vi "edittest List Sequences.vi"(6 "User Information":T1, 8 "error in (no error)":errorcluster, 10 "sxSequenceId (\"\")":string, 11 "Connection Refnum":T2) -> (0 "error out":errorcluster, 2 "Sequences List":string, 3 "Connection Refnum":T2)   [LabVIEW 2011]
uses:
  Summitek EXT/ODBC/SQL Controls/Connection Refnum.ctl
  server/database/Users/User Record.ctl
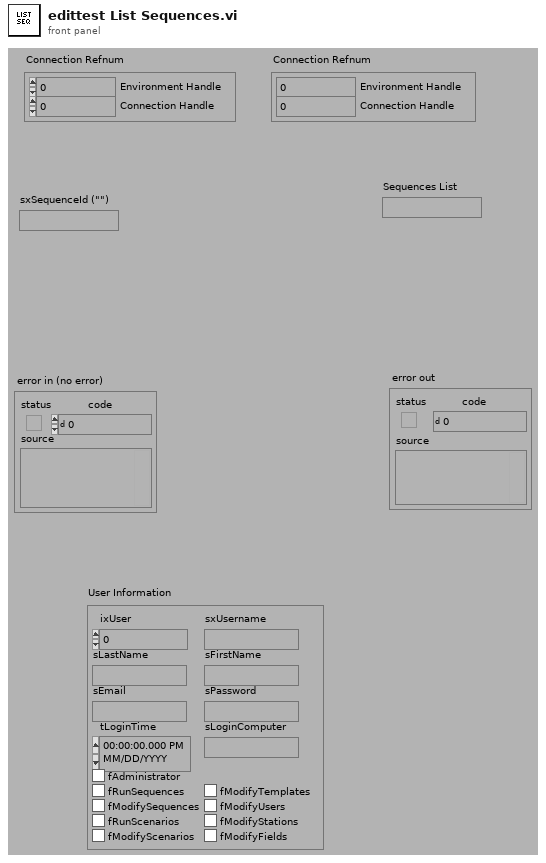
[diagram p1: front panel]
types:
  T1 = typedef "User Record.ctl" = cluster{"ixUser":i32, "sxUsername":string, "sLastName":string, "sFirstName":string, "sEmail":string, "sPassword":string, "tLoginTime":timestamp, "sLoginComputer":string, "fAdministrator":bool, "fRunSequences":bool, "fModifySequences":bool, "fRunScenarios":bool, "fModifyScenarios":bool, "fModifyTemplates":bool, "fModifyUsers":bool, "fModifyStations":bool, "fModifyFields":bool}
  T2 = typedef "Connection Refnum.ctl" = cluster{"Environment Handle":i32, "Connection Handle":i32}
  T3 = typedef "Sequence Record.ctl" = cluster{"ixSequence":i32, "sxSequenceId":string, "sDescription":string, "sCreator":string, "tCreationDate":timestamp, "sModifier":string, "tModifiedDate":timestamp, "fApproved":bool, "fSpartanSetsSN":bool, "fOverwriteData":bool, "fStopOnFail":bool, "fDisableQuickMode":bool, "fPartialExecution":bool, "fAutoNextItem":bool, "fDoNotPrintOnFail":bool}
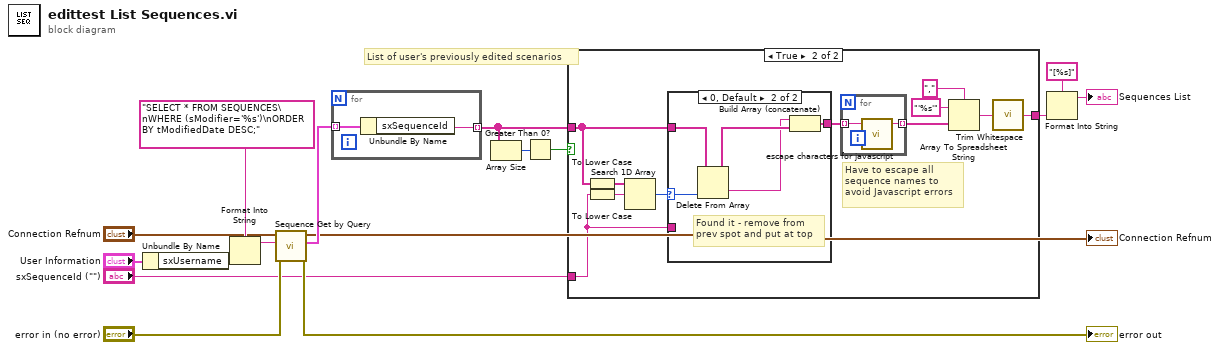
[diagram p0: block diagram]
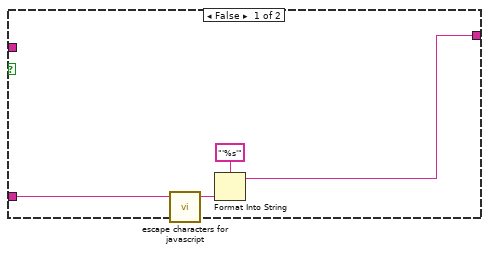
[diagram p2: hidden frame]
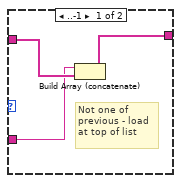
[diagram p3: hidden frame]
diagram:
  # "List of user's previously edited scenarios"
  n1 = Unbundle By Name("User Information") -> ("sxUsername"=w13:string)
  n2 = Format Into String(format string="SELECT * FROM SEQUENCES\nWHERE (sModifier='%s')\nORDER BY tModifiedDate DESC;", w13) -> (resulting string=w15:string)  [unwired: 2 in, 1 out]
  n3 = call "Sequence Get by Query.vi"("error in (no error)"="error in (no error)", "Sequence Query (\"\")"=w15, "Connection Refnum"="Connection Refnum") -> ("error out"=→"error out":errorcluster, "Records"=w14:T3[], "Connection Refnum"=→"Connection Refnum":T2)  [unwired: 6 out]
  n4 = for {
    tunnel: w14 -> [w18] mode=indexing
    tunnel: [w17] -> w2 mode=indexing
    n5 = Unbundle By Name(w18) -> ("sxSequenceId"=w17:string)
  }
  n6 = Array Size(array=w2) -> (size(s)=w6:i32)
  n7 = Greater Than 0?(x=w6) -> (x > 0?=w1:bool)
  n8 = case shown="True" w1 {
    tunnel: "sxSequenceId (\"\")" -> [w20 w25]
    tunnel: [w19 w27] -> w3
    tunnel: w2 -> [_ w26]
    frame False {
      n9 = call "escape characters for javascript.vi"("String (\"\")"=w20) -> ("escaped String"=w22:string)  [unwired: 4 out]
      n10 = Format Into String(format string="'%s'", w22) -> (resulting string=w19:string)  [unwired: 2 in, 1 out]
    }
    frame True {
      # "Have to escape all sequence names to avoid Javascript errors"
      n11 = To Lower Case(string=w26) -> (all lower case string=w28:string[])
      n12 = To Lower Case(string=w25) -> (all lower case string=w30:string)
      n13 = Search 1D Array(1D array=w28, element=w30) -> (index of element=w29:i32)  [unwired: 1 out]
      n14 = case shown="0, Default" w29 {
        selector: w29 -> [_ w42]
        tunnel: w26 -> [w38 w43]
        tunnel: w25 -> [w37 _]
        tunnel: [w36 w40] -> w23
        frame ..-1 {
          # "Not one of \nprevious - load\nat top of list"
          n15 = Build Array (concatenate)(w37, w38) -> (w36:string[])
        }
        frame 0, Default {
          # "Found it - remove from\nprev spot and put at top"
          n16 = Delete From Array(array=w43, index=w42) -> (deleted portion=w39:string, array with subset deleted=w41:string[])  [unwired: 1 in]
          n17 = Build Array (concatenate)(w39, w41) -> (w40:string[])
        }
      }
      n18 = for {
        tunnel: [w35] -> w24 mode=indexing
        tunnel: w23 -> [w34] mode=indexing
        n19 = call "escape characters for javascript.vi"("String (\"\")"=w34) -> ("escaped String"=w35:string)  [unwired: 4 out]
      }
      n20 = Array To Spreadsheet String(delimiter (Tab)=",", array=w24, 3:"'%s'") -> (spreadsheet string=w31:string)
      n21 = call <vilib>:"Trim Whitespace.vi"("string"=w31) -> ("trimmed string"=w27:string)  [unwired: 1 in]
    }
  }
  n22 = Format Into String(format string="[%s]", w3) -> (resulting string=→"Sequences List":string)  [unwired: 2 in, 1 out]
